vi "U3 Counter Config.vi"(8 "error in":errorcluster) -> (0 "error out":errorcluster)   [LabVIEW 2021]
panel:
  # "Enables both timers as firmware counters and enables both hardware counters.  FIO0-FIO3."
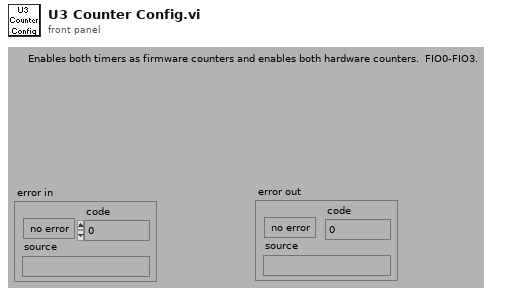
[diagram p1: front panel]
types:
  T1 = cluster{"Open LabJack":bool, "Address":string, "FirstFound":bool}
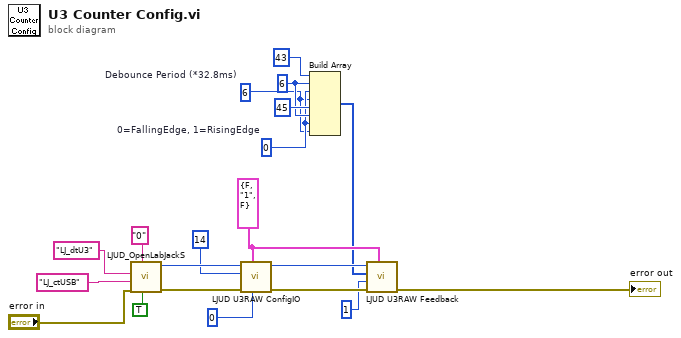
[diagram p0: block diagram]
diagram:
  w4 = u8 6  # Debounce Period (*32.8ms)
  w5 = u8 0  # 0=FallingEdge, 1=RisingEdge
  w8 = u8 6 ("Input Element")
  w12 = T1 {"Open LabJack"=FALSE, "Address"="1", "FirstFound"=FALSE} ("Comm Settings")
  n1 = call "LJUD_OpenLabJackS.vi"("FirstFound"=TRUE, "Address"="0", "error in"="error in", "ConnectionType"="LJ_ctUSB", "DeviceType"="LJ_dtU3") -> ("error out"=w15:errorcluster, "Handle"=w16:i32)  [unwired: 4 in, 1 out]
  n2 = call "LJUD U3RAW ConfigIO.vi"("FIOAnalog"=u8 0 ("FIODigital"), "Comm Settings"=w12, "error in (no error)"=w15, "WriteMask"=u8 14 ("TimerCounterEnable"), "Handle In"=w16) -> ("error out"=w11:errorcluster, "Handle Out"=w10:i32)  [unwired: 5 in]
  n3 = Build Array(u8 43 ("Input Element"), w8, w5, w4, u8 45 ("Input Element"), w8, w5, w4) -> (w7:u8[])
  n4 = call "LJUD U3RAW Feedback.vi"("Comm Settings"=w12, "error in (no error)"=w11, "# Data Bytes to Read"=1, "Data"=w7, "Handle In"=w10) -> ("error out"=→"error out":errorcluster)  [unwired: 4 in, 2 out]
